vi "connection_test.vi"() -> ()   [LabVIEW 2017]
uses:
  <vilib>/Plasmionique/MB Master/MB_Master_Serial/MB_Master_Serial.lvclass
  D:/Program Files (x86)/National Instruments/LabVIEW 2017/vi.lib/Plasmionique/MB Master/MB_Master/MB_Master.lvclass
  <vilib>/Plasmionique/MB Master/MB Master.lvlib
panel:
  out "Error out":errorcluster
  out "code":i32
  out "error":bool
  out "po":bool[](array[boolean])
  in  "Slave ID":u8=2
  out "przed wlaczeniem":bool[](array[boolean])
  in  "VISA Resource":refnum<visa-resource-name>="COM8"
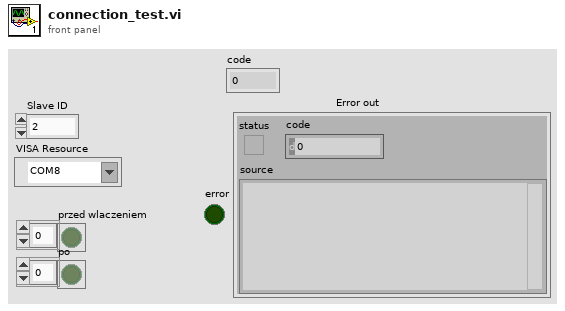
[diagram p1: front panel]
types:
  T1 = cluster{"baud rate (bps)":u32, "stop bits":u16, "parity":u16, "flow control":u16, "timeout":u32, "retries":i32}
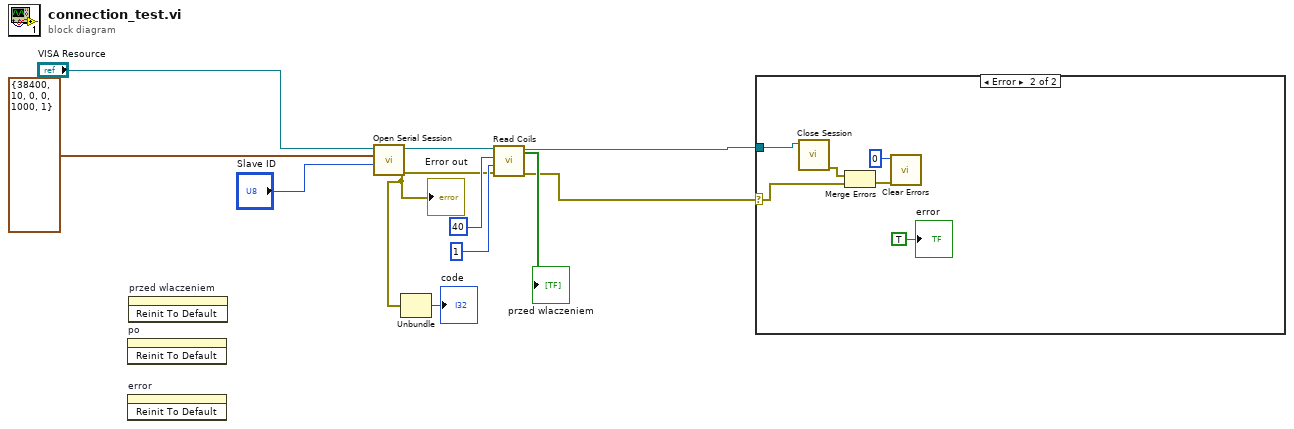
[diagram p0: block diagram]
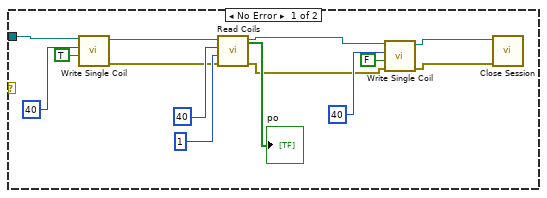
[diagram p2: hidden frame]
diagram:
  n1 = invoke on="po" class="Arr (strict)" method="Reinit To Default"() -> ()  [unwired: 3 in, 3 out]
  n2 = invoke on="error" class="Bool (strict)" method="Reinit To Default"() -> ()  [unwired: 3 in, 3 out]
  n3 = invoke on="przed wlaczeniem" class="Arr (strict)" method="Reinit To Default"() -> ()  [unwired: 3 in, 3 out]
  n4 = call <vilib>:"Open Serial Session.vi"("Slave ID"="Slave ID", "Serial Config"=T1 {"baud rate (bps)"=38400, "stop bits"=10, "parity"=0, "flow control"=0, "timeout"=1000, "retries"=1}, "VISA Resource"="VISA Resource") -> ("Error out"=w2:errorcluster, "MB_Serial session"=w5:refnum<class "MB_Master_Serial.lvclass">)  [unwired: 7 in]
  "Error out" <- w2
  n5 = Unbundle(w2) -> ("code"=→"code":i32)  [unwired: 2 out]
  n6 = call <vilib>:"Read Coils.vi"("error in (no error)"=w2, "quantity"=u16 1, "starting address"=u16 40, "MB session in"=w5) -> ("error out"=w3:errorcluster, "Coils"=→"przed wlaczeniem":bool[], "MB session out"=w4:refnum<class "MB_Master_Serial.lvclass">)  [unwired: 5 in]
  n7 = case shown="Error" w3 {
    selector: w3 -> [_ w29]
    tunnel: w4 -> [w22 w31]
    frame No Error {
      n8 = call <vilib>:"Write Single Coil.vi"("value"=TRUE, "address"=u16 40 ("starting address"), "MB session in"=w22) -> ("error out"=w21:errorcluster, "MB session out"=w20:refnum<class "MB_Master_Serial.lvclass">)  [unwired: 7 in]
      n9 = call <vilib>:"Read Coils.vi"("error in (no error)"=w21, "quantity"=u16 1, "starting address"=u16 40, "MB session in"=w20) -> ("error out"=w14:errorcluster, "Coils"=→"po":bool[], "MB session out"=w15:refnum<class "MB_Master_Serial.lvclass">)  [unwired: 5 in]
      n10 = call <vilib>:"Write Single Coil.vi"("error in (no error)"=w14, "value"=FALSE, "address"=u16 40 ("starting address"), "MB session in"=w15) -> ("error out"=w13:errorcluster, "MB session out"=w12:refnum<class "MB_Master_Serial.lvclass">)  [unwired: 6 in]
      n11 = call-dynamic "Close Session.vi"("error in (no error)"=w13, "MB_Serial session"=w12) -> ()  [unwired: 9 in, 1 out]
    }
    frame Error {
      n12 = call-dynamic "Close Session.vi"("MB_Serial session"=w31) -> ("error out"=w30:errorcluster)  [unwired: 10 in]
      n13 = Merge Errors(w30, w29) -> (w28:errorcluster)
      n14 = call <vilib>:"Clear Errors.vi"("error in (no error)"=w28, "specific error code to clear (0: all)"=0) -> ()  [unwired: 4 in, 2 out]
      "error" <- TRUE ("error")
    }
  }
